vi "Build Status Broadcast Message.vi"(5 "State With Arguments":string, 7 "Arguments (\"\")":string) -> (6 "CSM Message String":string)   [LabVIEW 2017, in "Communicable State Machine.lvlib"]
doc: "Concatenates normal status message strings. The message format is as follows:\n\n Status >> Arguments -><status>\n // The following strings are equivalent operations.\n // More operation characters are defined for easier typing and memorization.\n Status >> Arguments -><broadcast>\n Status >> Arguments -><all>\n\n\n> [!NOTE] <b>Message Building API</b>\n>\n> This type of API is only used to concatenate message strings and does not send messages directly. The strings need to be merged into the CSM state queue, and the messages will be sent and the operation executed within the Parse State Queue++ VI. If you are familiar with CSM rules, you do not need to use this type of API. You can type the corresponding message string or operation string directly into the string.\n\n\n-- <b>Controls</b> --\n- <b>State with Arguments</b>: CSM normal status message string.\n- <b>Arguments (\"\")</b>: Argument information. Arguments contained in <b>State with Arguments</b> will be replaced.\n\n-- <b>Indicators</b> --\n- <b>CSM Message String</b>: Concatenated CSM message string."
uses:
  Communicable State Machine.lvlib
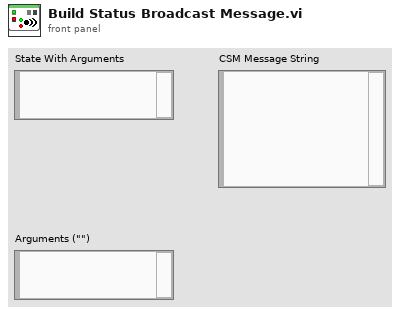
[diagram p1: front panel]
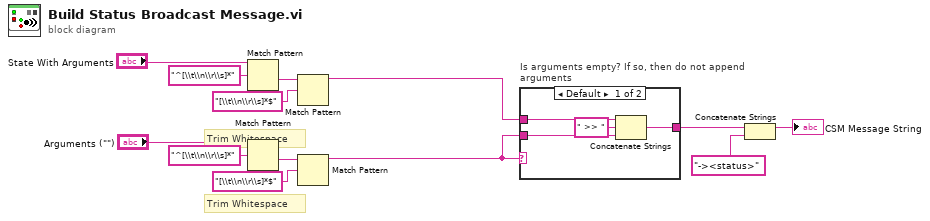
[diagram p0: block diagram]
diagram:
  # "Trim Whitespace"
  # "Trim Whitespace"
  n1 = Match Pattern(string="State With Arguments", regular expression="^[\\t\\n\\r\\s]*") -> (after substring=w4:string)  [unwired: 1 in, 3 out]
  n2 = Match Pattern(string="Arguments (\"\")", regular expression="^[\\t\\n\\r\\s]*") -> (after substring=w12:string)  [unwired: 1 in, 3 out]
  n3 = Match Pattern(string=w4, regular expression="[\\t\\n\\r\\s]*$") -> (before substring=w1:string)  [unwired: 1 in, 3 out]
  n4 = Match Pattern(string=w12, regular expression="[\\t\\n\\r\\s]*$") -> (before substring=w7:string)  [unwired: 1 in, 3 out]
  n5 = case "Is arguments empty? If so, then do not append arguments" shown="Default" w7 {
    tunnel: [w14 w18] -> w8
    tunnel: w1 -> [w17 w18]
    tunnel: w7 -> [w15 _]
    frame Default {
      n6 = Concatenate Strings(w17, " >> " ("string"), w15) -> (w14:string)
    }
    frame "" {
    }
  }
  n7 = Concatenate Strings(w8, "-><status>" ("string")) -> (→"CSM Message String":string)
